vi "Move Snake.vi"(7 "Packed refs":T1, 8 "error in (no error)":errorcluster, 10 "Direction":T2, 11 "Board Game in":refnum<class "Board Game.lvclass">) -> (0 "error out":errorcluster, 3 "Board Game out":refnum<class "Board Game.lvclass">)   [LabVIEW 2021, in "Board Game.lvclass"]
uses:
  Board Game.lvclass
  Board Game.lvclass/Board Game.ctl
  GameEl_class/GameEl.lvclass
  Shield/Shield.lvclass
  Snake_class/Snake.lvclass
  C:/Users/poche/Programs/LabVIEW/imposible snake/GameEl_class/GameEl.lvclass
  C:/Users/poche/Programs/LabVIEW/imposible snake/Snake_class/Snake.lvclass
  GameEl_class/private/Enum Direction.ctl
  LVApp/Modules/Sound Manager/Typedefs/Sound Effects.ctl
  Application/Packed Refs.ctl
  Application/Application.lvclass
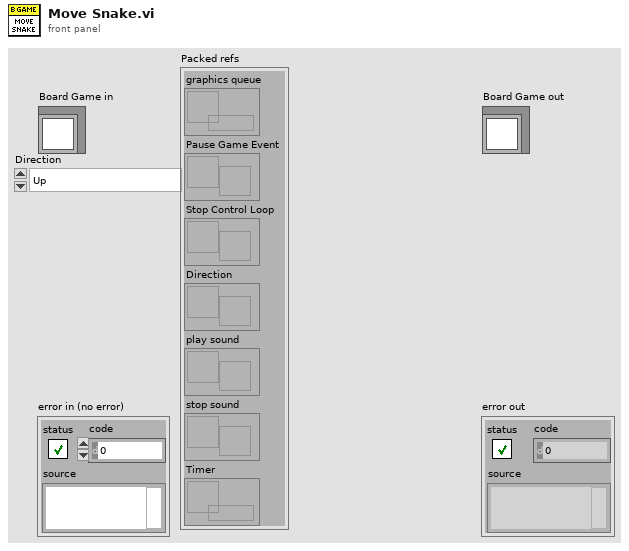
[diagram p1: front panel]
types:
  T1 = typedef "Application.lvclass/Packed Refs.ctl" = cluster{"graphics queue":refnum<queue>, "Pause Game Event":refnum<user-event>, "Stop Control Loop":refnum<user-event>, "Direction":refnum<notifier>, "play sound":refnum<user-event>, "stop sound":refnum<user-event>, "Timer":refnum<data-value>}
  T2 = typedef "GameEl.lvclass/Enum Direction.ctl" = enum16{"Up", "Down", "Forward", "Backward"}
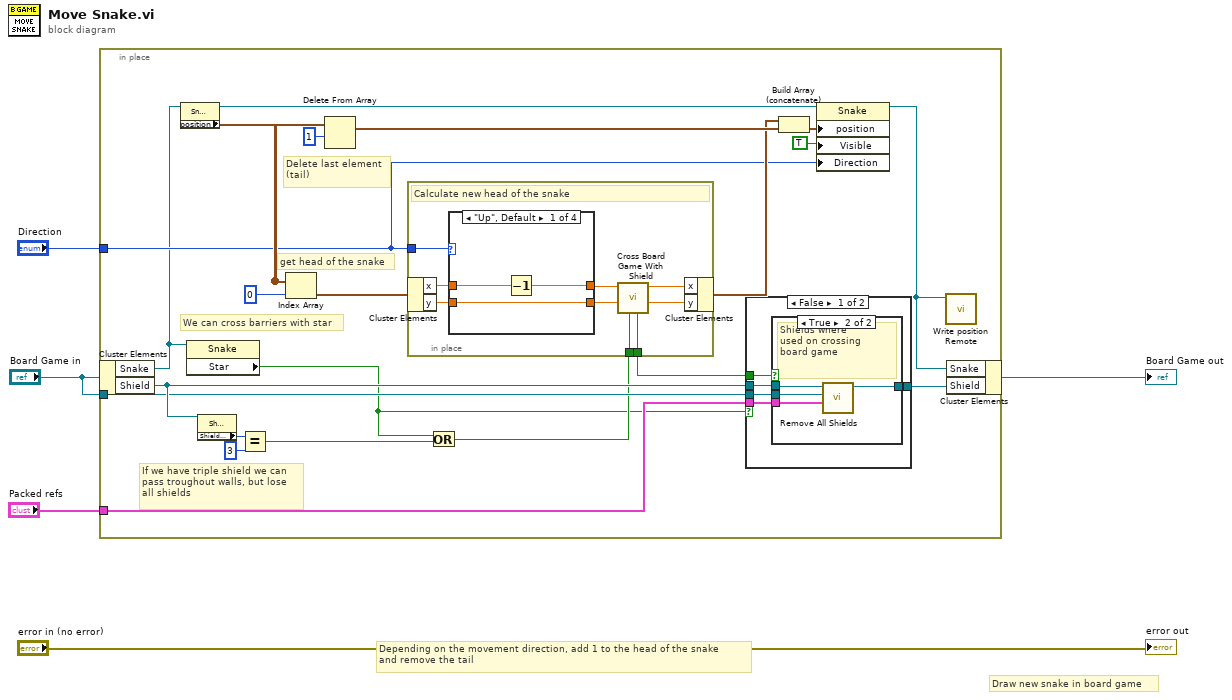
[diagram p0: block diagram]
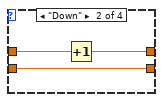
[diagram p4: hidden frame]
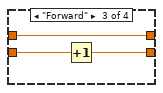
[diagram p5: hidden frame]
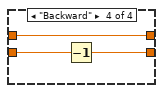
[diagram p6: hidden frame]
diagram:
  # "Draw new snake in board game"
  # "Depending on the movement direction, add 1 to the head of the snake\nand remove the tail"
  n1 = in-place {
    in-place-border: "Direction" -> [w9]
    in-place-border: "Packed refs" -> [w10]
    in-place-border: "Board Game in" -> [w11]
    # "We can cross barriers with star"
    # "If we have triple shield we can\npass troughout walls, but lose \nall shields"
    # "get head of the snake"
    # "Delete last element \n(tail)"
    n2 = in-place-cluster #1("Board Game in") -> ("Snake"=w7:refnum<class "Snake.lvclass">, "Shield"=w13:refnum<class "Shield.lvclass">)
    n3 = property class="Snake"(reference=w7) -> (reference out=w15:refnum<class "Snake.lvclass">, "position"=w25:cluster{"x":dbl, "y":dbl}[])  [unwired: 1 in, 1 out]
    n4 = property class="Snake"(reference=w7) -> ("Star"=w6:bool)  [unwired: 1 in, 2 out]
    n5 = property class="Shield.lvclass"(reference=w13) -> ("Shield Count"=w18:u8)  [unwired: 1 in, 2 out]
    n6 = Equal?(x=w18, y=u8 3) -> (x = y?=w16:bool)
    n7 = Index Array(array=w25, index=0) -> (element=w23:cluster{"x":dbl, "y":dbl})
    n8 = Delete From Array(array=w25, length=1) -> (array with subset deleted=w26:cluster{"x":dbl, "y":dbl}[])  [unwired: 1 in, 1 out]
    n9 = Or(x=w6, y=w16) -> (x .or. y?=w8:bool)
    n10 = in-place {
      in-place-border: w9 -> [w47]
      in-place-border: w8 -> [w44]
      in-place-border: [w39] -> w14
      # "Calculate new head of the snake"
      n11 = in-place-cluster #2(w23) -> ("x"=w46:dbl, "y"=w45:dbl)
      n12 = case shown="\"Up\", Default" w47 {
        tunnel: w46 -> [w50 w53 w56 w59]
        tunnel: w45 -> [w49 w52 w55 w58]
        tunnel: [w48 w51 w56 w59] -> w43
        tunnel: [w49 w52 w54 w57] -> w42
        frame "Up", Default {
          n13 = Decrement(x=w50) -> (x-1=w48:dbl)
        }
        frame "Down" {
          n14 = Increment(x=w53) -> (x+1=w51:dbl)
        }
        frame "Forward" {
          n15 = Increment(x=w55) -> (x+1=w54:dbl)
        }
        frame "Backward" {
          n16 = Decrement(x=w58) -> (x-1=w57:dbl)
        }
      }
      n17 = call "Cross Board Game With Shield.vi"("Max Shield?"=w44, "y"=w42, "x"=w43) -> ("y out"=w40:dbl, "x out"=w41:dbl, "Crossed?"=w39:bool)  [unwired: 6 in]
      n18 = in-place-cluster #2("x"=w41, "y"=w40) -> (w22:cluster{"x":dbl, "y":dbl})
    }
    n19 = case shown="False" w6 {
      tunnel: w14 -> [w32 _]
      tunnel: w13 -> [w31 w38]
      tunnel: [w30 w38] -> w12
      tunnel: w11 -> [w29 _]
      tunnel: w10 -> [w28 _]
      frame False {
        n20 = case shown="True" w32 {
          tunnel: w31 -> [w33 w37]
          tunnel: [w33 w36] -> w30
          tunnel: w29 -> [_ w35]
          tunnel: w28 -> [_ w34]
          frame False {
          }
          frame True {
            # "Shields where\nused on crossing\nboard game"
            n21 = call "Remove All Shields.vi"("Packed refs"=w34, "Board Game in"=w35, "Shield in"=w37) -> ("Shield out"=w36:refnum<class "Shield.lvclass">)  [unwired: 7 in, 1 out]
          }
        }
      }
      frame True {
      }
    }
    n22 = Build Array (concatenate)(w22, w26) -> (w21:cluster{"x":dbl, "y":dbl}[])
    n23 = property class="Snake"(reference=w15, "position"=w21, "Visible"=TRUE, "Direction"=w9) -> (reference out=w20:refnum<class "Snake.lvclass">)  [unwired: 1 in, 1 out]
    n24 = call "Write position Remote.vi"("GameEl in"=w20) -> ()  [unwired: 10 in, 1 out]
    n25 = in-place-cluster #1("Snake"=w20, "Shield"=w12) -> (→"Board Game out":refnum<class "Board Game.lvclass">)
  }
  "error out" <- "error in (no error)"
